vi "TRIG_AUX_COUN.vi"(0 "VISA IN":refnum<visa-resource-name>, 5 "error in":errorcluster) -> (14 "VISA Out":refnum<visa-resource-name>, 19 "error out":errorcluster)   [LabVIEW 2018, in "PNA-X.lvlib"]
doc: "TRIGger:AUX:COUNt? \n(Read-only) Returns the number of AUX trigger input / output connector pairs in the instrument. \nPNA-X = 2 \nE836xB and PNA-L models = 1 \nParameters \nExamples TRIG:CHAN:AUX:COUN? \ntrigger:channel2:aux:count? \nReturn Type Numeric \nDefault Not Applicable"
uses:
  PNA-X.lvlib
panel:
  out "Data":i32
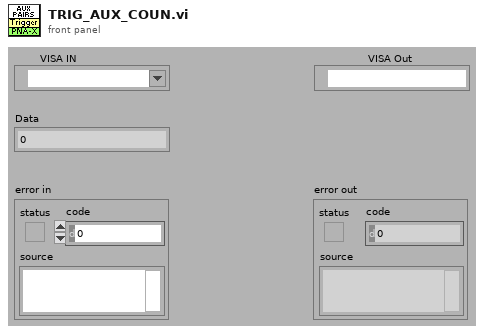
[diagram p1: front panel]
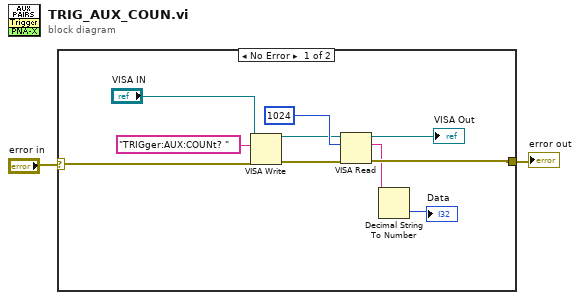
[diagram p0: block diagram]
diagram:
  n1 = case shown="No Error" "error in" {
    selector: "error in" -> [w4 w13]
    tunnel: [w7 w13] -> w1
    frame No Error {
      n2 = VISA Write(VISA resource name="VISA IN", write buffer="TRIGger:AUX:COUNt? " ("Cmdline"), error in (no error)=w4) -> (VISA resource name out=w9:refnum<visa-resource-name>, error out=w11:errorcluster)  [unwired: 1 out]
      n3 = VISA Read(VISA resource name=w9, byte count=1024, error in (no error)=w11) -> (VISA resource name out=→"VISA Out":refnum<visa-resource-name>, read buffer=w6:string, error out=w7:errorcluster)  [unwired: 1 out]
      n4 = Decimal String To Number(string=w6) -> (number=→"Data":i32)  [unwired: 2 in, 1 out]
    }
    frame Error {
    }
  }
  "error out" <- w1
